vi "Capture Matrix From String.vi"(11 "String":string) -> (3 "Matrix":i32[][](array[numeric]))   [LabVIEW 2019, in "Day 4.lvlib"]
uses:
  Day 4.lvlib
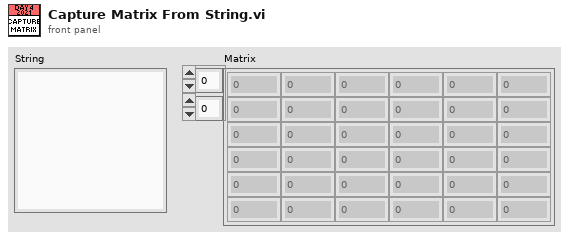
[diagram p1: front panel]
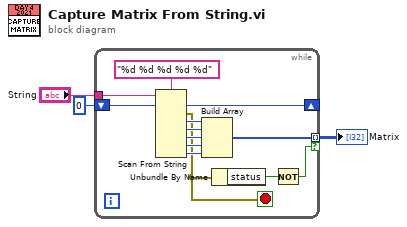
[diagram p0: block diagram]
diagram:
  n1 = while {
    tunnel: "String" -> [w15]
    tunnel: [w9] -> w3 mode=indexing if=w6
    shift-right: [w5] -> _
    shift-left: u32 0 -> [w4]
    stop <- w7 stop-if-true
    n2 = Scan From String(format string="%d %d %d %d %d", input string=w15, initial scan location=w4) -> (offset past scan=w5:u32, error out=w7:errorcluster, output 1=w14:i32, output 2=w13:i32, output 3=w12:i32, output 4=w11:i32, output 5=w10:i32)  [unwired: 6 in, 1 out]
    n3 = Build Array(w14, w13, w12, w11, w10) -> (w9:i32[])
    n4 = Unbundle By Name(w7) -> ("status"=w8:bool)
    n5 = Not(x=w8) -> (.not. x?=w6:bool)
  }
  "Matrix" <- w3
